vi "getRegExValue.vi"(7 "Name":string, 8 "error in (no error)":errorcluster, 11 "tBSONDocument in":refnum<class "tBSONDocument.lvclass">) -> (0 "error out":errorcluster, 1 "Options":T1, 2 "RegEx":string, 3 "tBSONDocument out":refnum<class "tBSONDocument.lvclass">)   [LabVIEW 2013, in "BSON.lvlib" / "tBSONDocument.lvclass"]
doc: "Retrieves a regular expression from a BSON document."
uses:
  tBSONDocument.lvclass
  BSONElements/tBSONRegEx/options.ctl
  BSONElements/tBSONRegEx/tBSONRegEx.lvclass
  BSONElements/tBSONRegEx/getRegularExpression.vi
  BSONElements/tBSONRegEx/getOptions.vi
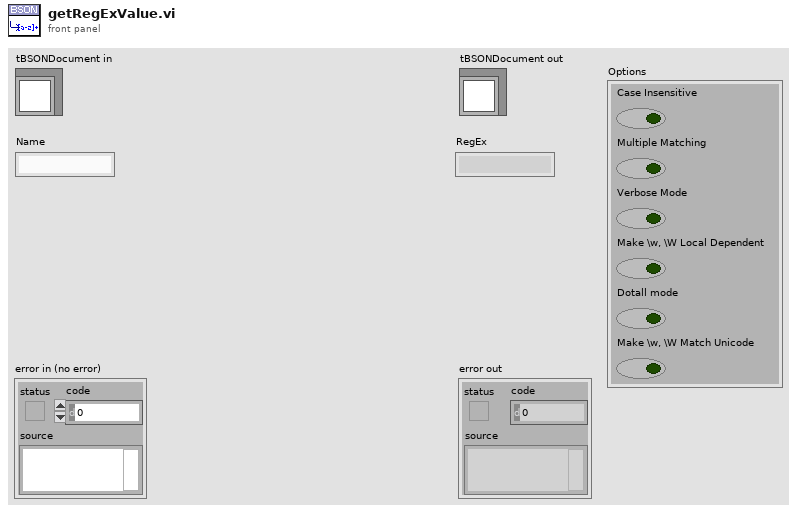
[diagram p1: front panel]
types:
  T1 = typedef "BSON.lvlib/tBSONRegEx.lvclass/options.ctl" = cluster{"Case Insensitive":bool, "Multiple Matching":bool, "Verbose Mode":bool, "Make \\w, \\W Local Dependent":bool, "Dotall mode":bool, "Make \\w, \\W Match Unicode":bool}
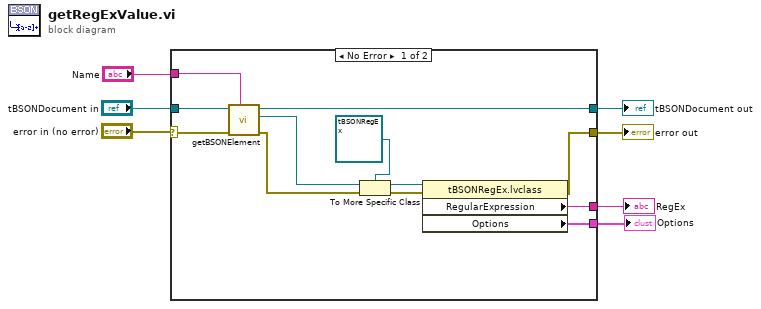
[diagram p0: block diagram]
diagram:
  n1 = case shown="No Error" "error in (no error)" {
    selector: "error in (no error)" -> [w18 w21]
    tunnel: [w12 w21] -> w3
    tunnel: [w13 w20] -> w4
    tunnel: "tBSONDocument in" -> [w19 w20]
    tunnel: "Name" -> [w10 _]
    tunnel: [w11 _] -> w2
    tunnel: [w8 _] -> w1
    frame No Error {
      n2 = call "getBSONElement.vi"("Name"=w10, "error in (no error)"=w18, "tBSONDocument in"=w19) -> ("error out"=w14:errorcluster, "Element"=w15:refnum<class "tBSONElement.lvclass">, "tBSONDocument out"=w13:refnum<class "tBSONDocument.lvclass">)  [unwired: 6 in]
      n3 = To More Specific Class(target class=refnum<class "tBSONRegEx.lvclass"> refnum ("lvMongoDriver.lvlib:BSON.lvlib:tBSONRegEx.lvclass"), reference=w15, error in=w14) -> (specific class reference=w17:refnum<class "tBSONRegEx.lvclass">, error out=w16:errorcluster)
      n4 = property class="tBSONRegEx.lvclass"(reference=w17, error in=w16) -> (error out=w12:errorcluster, "RegularExpression"=w11:string, "Options"=w8:T1)  [unwired: 1 out]
    }
    frame Error {
    }
  }
  "error out" <- w3
  "tBSONDocument out" <- w4
  "RegEx" <- w2
  "Options" <- w1
